vi "Utility - Update String with Error Cluster.vi"(8 "error in (no error)":errorcluster, 11 "String In":string) -> (0 "error out":errorcluster, 3 "String Out":string)   [LabVIEW 2014]
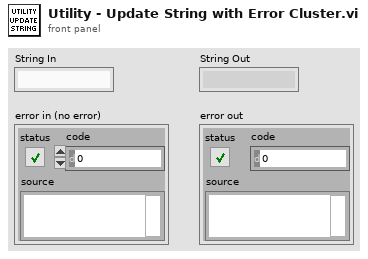
[diagram p1: front panel]
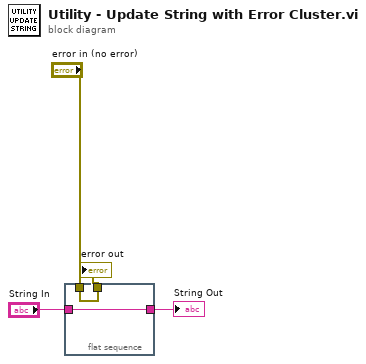
[diagram p0: block diagram]
diagram:
  n1 = flat-sequence {
    tunnel: "error in (no error)" -> [w5]
    tunnel: "String In" -> [w6]
    tunnel: [w6] -> w2
    tunnel: [w5] -> w4
    frame #0 {
    }
  }
  "error out" <- w4
  "String Out" <- w2
